vi "gen_semnal.vi"() -> ()   [LabVIEW 2009]
uses:
  <vilib>/Platform/portaccess.llb/Out Port8.vi
  <vilib>/Platform/portaccess.llb/In Port8.vi
panel:
  out "Waveform Graph":u32[](graph)
  out "Numeric":dbl
  in  "stop":bool
  out "Waveform Chart":u32(graph)
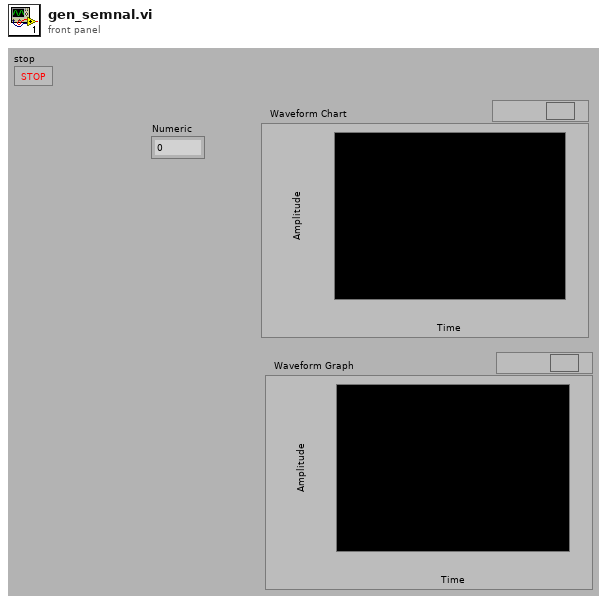
[diagram p1: front panel]
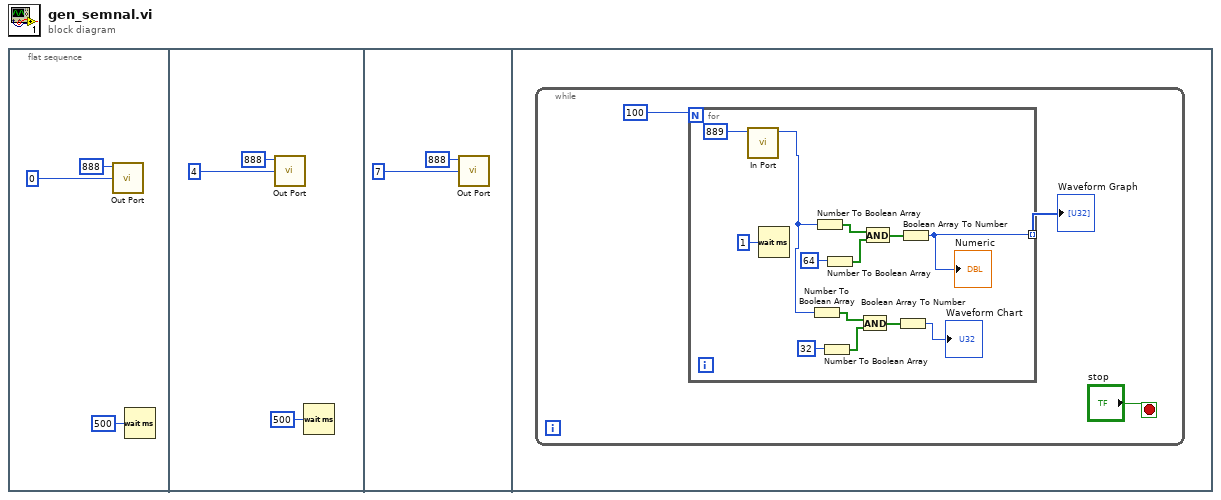
[diagram p0: block diagram]
diagram:
  n1 = flat-sequence {
    frame #0 {
      n2 = call-poly <vilib>:"Out Port.vi"("write value"=u8 0, "address"=i16 888) -> ()  [unwired: 7 in, 1 out]
      n3 = Wait (ms)(milliseconds to wait=u32 500) -> ()  [unwired: 1 out]
    }
    frame #1 {
      n4 = call-poly <vilib>:"Out Port.vi"("write value"=u8 4, "address"=i16 888) -> ()  [unwired: 7 in, 1 out]
      n5 = Wait (ms)(milliseconds to wait=u32 500) -> ()  [unwired: 1 out]
    }
    frame #2 {
      n6 = call-poly <vilib>:"Out Port.vi"("write value"=u8 7, "address"=i16 888) -> ()  [unwired: 7 in, 1 out]
    }
    frame #3 {
      n7 = while {
        stop <- "stop" stop-if-true
        n8 = for {
          N: 100 -> [_]
          tunnel: [w18] -> w9 mode=indexing
          n9 = call-poly <vilib>:"In Port.vi"("address"=i16 889) -> ("data read"=w12:i8)  [unwired: 7 in, 1 out]
          n10 = Wait (ms)(milliseconds to wait=u32 1) -> ()  [unwired: 1 out]
          n11 = Number To Boolean Array(number=w12) -> (Boolean array=w17:bool[])
          n12 = Number To Boolean Array(number=w12) -> (Boolean array=w22:bool[])
          n13 = Number To Boolean Array(number=u32 32 ("milliseconds to wait")) -> (Boolean array=w15:bool[])
          n14 = Number To Boolean Array(number=u32 64 ("milliseconds to wait")) -> (Boolean array=w20:bool[])
          n15 = And(x=w17, y=w15) -> (x .and. y?=w14:bool[])
          n16 = And(x=w22, y=w20) -> (x .and. y?=w19:bool[])
          n17 = Boolean Array To Number(Boolean array=w14) -> (number=→"Waveform Chart":u32)
          n18 = Boolean Array To Number(Boolean array=w19) -> (number=w18:u32)
          "Numeric" <- w18
        }
        "Waveform Graph" <- w9
      }
    }
  }
